vi "Set Defaults.vi"(11 "NewEntityTemplate in":refnum<class "LiveDemo.lvclass">) -> (3 "NewEntityTemplate out":refnum<class "LiveDemo.lvclass">)   [LabVIEW 2020, in "tests.lvlib" / "LiveDemo.lvclass"]
uses:
  LiveDemo.lvclass
  LiveDemo.lvclass/LiveDemo.ctl
  <vilib>/IlluminatedG/IG Conditum Base/Conditum/Columns/Boolean/Boolean.lvclass
  <vilib>/IlluminatedG/IG Conditum Base/Conditum/Columns/Double/Double.lvclass
  <vilib>/IlluminatedG/IG Conditum Base/Conditum/Columns/String/String.lvclass
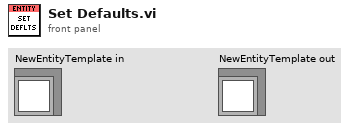
[diagram p1: front panel]
types:
  T1 = typedef "tests.lvlib/LiveDemo.lvclass/Columns.ctl" = cluster{"Active":refnum<class "Boolean.lvclass">, "Score":refnum<class "Double.lvclass">, "Name":refnum<class "String.lvclass">}
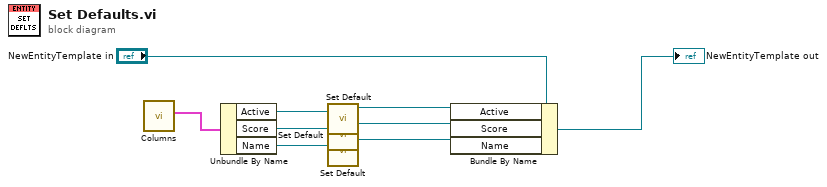
[diagram p0: block diagram]
diagram:
  n1 = call "Columns.vi"() -> ("Columns"=w7:T1)  [unwired: 11 in]
  n2 = Unbundle By Name(w7) -> ("Active"=w6:refnum<class "Boolean.lvclass">, "Score"=w5:refnum<class "Double.lvclass">, "Name"=w4:refnum<class "String.lvclass">)
  n3 = call-dynamic "Set Default.vi"("Boolean in"=w6) -> ("Boolean out"=w3:refnum<class "Boolean.lvclass">)  [unwired: 10 in]
  n4 = call-dynamic "Set Default.vi"("Double in"=w5) -> ("Double out"=w2:refnum<class "Double.lvclass">)  [unwired: 10 in]
  n5 = call-dynamic "Set Default.vi"("String in"=w4) -> ("String out"=w1:refnum<class "String.lvclass">)  [unwired: 10 in]
  n6 = Bundle By Name(cluster="NewEntityTemplate in", "Active"=w3, "Score"=w2, "Name"=w1) -> (→"NewEntityTemplate out":refnum<class "LiveDemo.lvclass">)
